vi "Test Variant to JSON TMP.vi"() -> ()   [LabVIEW 2011]
uses:
  JSON Scalar/Infinity&NaN.ctl
  JSON Value/JSON Value.lvclass
  Variant JSON.lvlib
  JSON Scalar/JSON Scalar.lvclass
panel:
  in  "Treatment of Infinity/NaN":T1
  in  "Test Cluster":T2={"T2"="test2", "T1"=456.789, "Nest"={"Enum"=enum."AAA", "NestNest"={"A"="Hi", "B"=2.0, "C"=1}}, "Test Array"=[456.789, 2.0, 3.0], "Boolean"=FALSE}
  out "JSON String":string
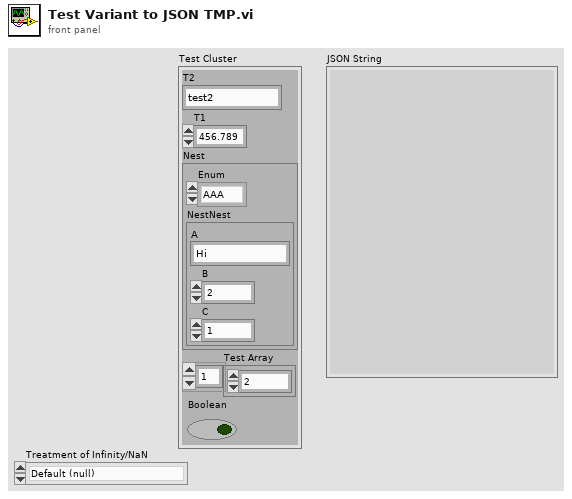
[diagram p1: front panel]
types:
  T1 = typedef "JSON Scalar.lvclass/Infinity&NaN.ctl" = enum16{"Default (null)", "Extended", "LabVIEW extensions"}
  T2 = cluster{"T2":string, "T1":dbl, "Nest":cluster{"Enum":enum16{"AAA", "BBB", "CCC"}, "NestNest":cluster{"A":string, "B":dbl, "C":i16}}, "Test Array":dbl[], "Boolean":bool}
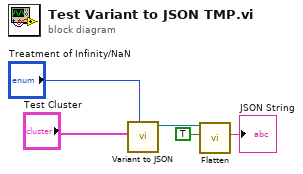
[diagram p0: block diagram]
diagram:
  n1 = call "Variant to JSON.vi"("Treatment of Infinity/NaN"="Treatment of Infinity/NaN", "Variant"="Test Cluster") -> ("JSON Value out"=w3:refnum<class "JSON Value.lvclass">)  [unwired: 8 in, 1 out]
  n2 = call-dynamic "Flatten.vi"("Pretty Print?"=TRUE, "JSON Value in"=w3) -> ("String"=→"JSON String":string)  [unwired: 8 in, 1 out]
